vi "Change Output Setpoint.vi"() -> ()   [LabVIEW 2020]
uses:
  <vilib>/Skyline/Tag/Shared/typedefs/DataType.ctl
  <vilib>/Skyline/Tag/Wrapper/Wrapper AMQP_class/Open Tag AMQP.vi
  <vilib>/Skyline/Tag/Wrapper/Wrapper_class/Write Tag (DBL).vi
  <vilib>/Skyline/Tag/Wrapper/Wrapper_class/Close Tag (Single).vi
  <vilib>/Skyline/Tag/Wrapper/Wrapper_class/NI Skyline Tag.lvclass
  <vilib>/Skyline/Tag/Wrapper/Wrapper AMQP_class/NI Skyline Tag AMQP.lvclass
  <vilib>/Skyline/Tag/Shared/NI Skyline Tag.lvlib
  FlexLoggerTagHelpers.lvlib
panel:
  in  "Channel value":dbl
  in  "Channel name":string
  # "Overview: This is example changes the value of the setpoint for an output in FlexLogger\nRequirements: LabVIEW Full Development System, FlexLogger\nInstructions:\n1. Launch FlexLogger\n     a. Create a Project\n     b. Configure one or more output channels in the Channel Specification\n2. Specify the channel name and value of the setpoint to change on the front panel of this VI.    \n2. Run this VI\n3. Note that the setpoint of the channel in FlexLogger changes to the value specified"
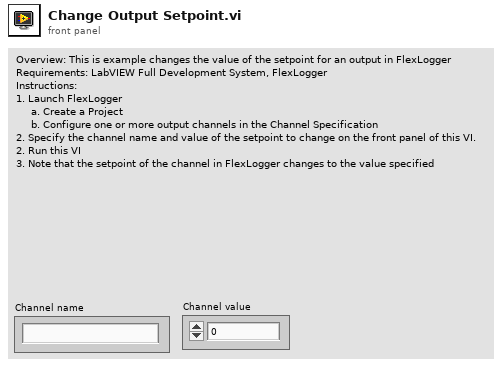
[diagram p1: front panel]
types:
  T1 = typedef "NI Skyline Tag.lvlib/DataType.ctl" = enum32{"Double", "I32", "String", "Boolean", "U64", "Timestamp"}
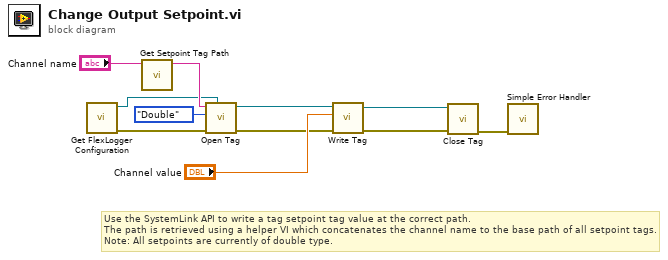
[diagram p0: block diagram]
diagram:
  # "Use the SystemLink API to write a tag setpoint tag value at the correct path.\nThe path is retrieved using a helper VI which concatenates the channel name to the base path of all setpoint tags.  \nNote: All setpoints are currently of double type."
  n1 = call "Get FlexLogger Configuration.vi"() -> ("error out"=w2:errorcluster, "Local FlexLogger Configuration"=w1:refnum<class "NI Skyline Configuration AMQP.lvclass">)  [unwired: 10 in]
  n2 = call "Get Setpoint Tag Path.vi"("channel Name"="Channel name") -> ("tag path"=w3:string)  [unwired: 10 in]
  n3 = call-poly <vilib>:"Open Tag.vi"("configuration"=w1, "error in (no error)"=w2, "data type"=DataType."Double", "path"=w3) -> ("error out"=w5:errorcluster, "tag"=w10:refnum<class "NI Skyline Tag.lvclass">)  [unwired: 6 in]
  n4 = call-poly <vilib>:"Write Tag.vi"("error in (no error)"=w5, "value"="Channel value", "tag in"=w10) -> ("error out"=w7:errorcluster, "tag out"=w8:refnum<class "NI Skyline Tag.lvclass">)  [unwired: 7 in]
  n5 = call-poly <vilib>:"Close Tag.vi"("error in (no error)"=w7, "tag"=w8) -> ("error out"=w6:errorcluster)  [unwired: 9 in]
  n6 = call <vilib>:"Simple Error Handler.vi"("error in (no error)"=w6) -> ()  [unwired: 4 in, 5 out]
